vi "Encontrar Fila del Qr en Sheets.vi"(11 "QR":string) -> (2 "hora_entrada":timestamp, 3 "indice del QR":i32)   [LabVIEW 2025]
uses:
  <vilib>/httpClient/LabVIEWHTTPClient.lvlib
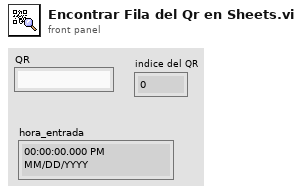
[diagram p1: front panel]
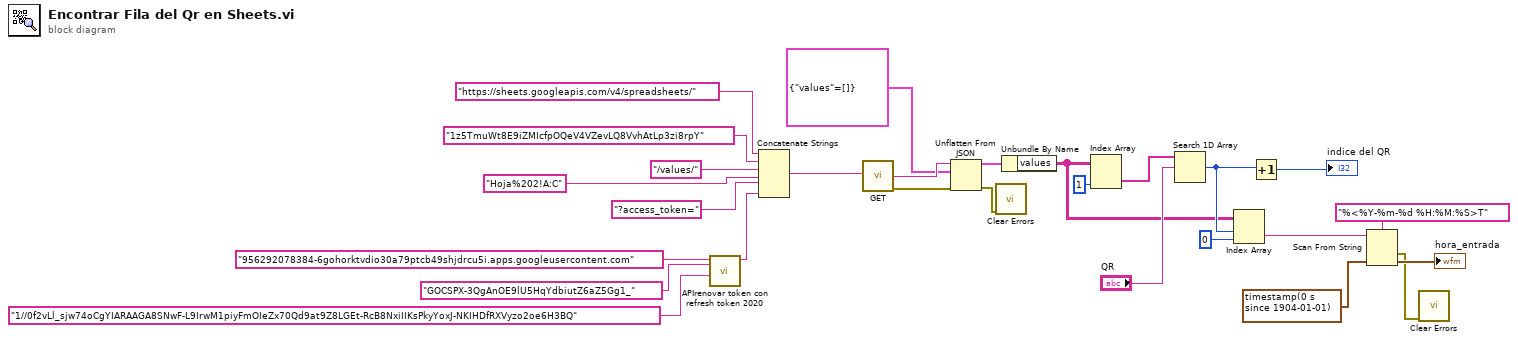
[diagram p0: block diagram]
diagram:
  n1 = call "APIrenovar token con refresh token 2020.vi"("refresh_token"="1//0f2vLl_sjw74oCgYIARAAGA8SNwF-L9IrwM1piyFmOIeZx70Qd9at9Z8LGEt-RcB8NxiIIKsPkyYoxJ-NKIHDfRXVyzo2oe6H3BQ", "client_secret"="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", "client_id"="956292078384-6gohorktvdio30a79ptcb49shjdrcu5i.apps.googleusercontent.com") -> ("access_token"=w12:string)  [unwired: 8 in]
  n2 = Concatenate Strings("https://sheets.googleapis.com/v4/spreadsheets/", "1z5TmuWt8E9iZMIcfpOQeV4VZevLQ8VvhAtLp3zi8rpY" ("spreadsheet_id"), "/values/", "Hoja%202!A:C" ("write_range"), "?access_token=", w12) -> (w11:string)
  n3 = call <vilib>:"GET.vi"("url"=w11) -> ("body"=w27:string, "error out"=w25:errorcluster)  [unwired: 11 in, 2 out]
  n4 = Unflatten From JSON(JSON string=w27, type and defaults=cluster{"values":string[][]} {"values"=[]}, error in (no error)=w25) -> (value=w24:cluster{"values":string[][]}, error out=w10:errorcluster)  [unwired: 4 in]
  n5 = call <vilib>:"Clear Errors.vi"("error in (no error)"=w10) -> ()  [unwired: 5 in, 2 out]
  n6 = Unbundle By Name(w24) -> ("values"=w8:string[][])
  n7 = Index Array(array=w8, index (col)=1 ("index")) -> (element=w22:string[])  [unwired: 1 in]
  n8 = Search 1D Array(1D array=w22, element="QR") -> (index of element=w9:i32)  [unwired: 1 in]
  n9 = Index Array(array=w8, index (row)=w9, index (col)=0 ("index")) -> (element=w6:string)
  n10 = Increment(x=w9) -> (x+1=→"indice del QR":i32)
  n11 = Scan From String(format string="%<%Y-%m-%d %H:%M:%S>T", input string=w6, default 1=timestamp(0 s since 1904-01-01)) -> (error out=w1:errorcluster, output 1=→"hora_entrada":timestamp)  [unwired: 2 in, 2 out]
  n12 = call <vilib>:"Clear Errors.vi"("error in (no error)"=w1) -> ()  [unwired: 5 in, 2 out]
